vi "Lvi Read Dbl Data Pt.vi"(8 "error in (no error)":errorcluster, 10 "timeout":dbl, 11 "TaskRef":i32) -> (0 "error out":errorcluster, 1 "function return":i32, 2 "DataBuf":dbl, 3 "TaskRef out":i32)   [LabVIEW 2016, in "DtLvLink.lvlib"]
doc: "Calls directly into the entry points of the DLL of the Data Acq SDK to return data points (double data type) from the specified task. This VI is used by the higher-level VI, DtOLRead."
uses:
  <userlib>/LV-Link3/DtLvLink.lvlib
  <userlib>/LV-Link3/DtLvLink_32.dll
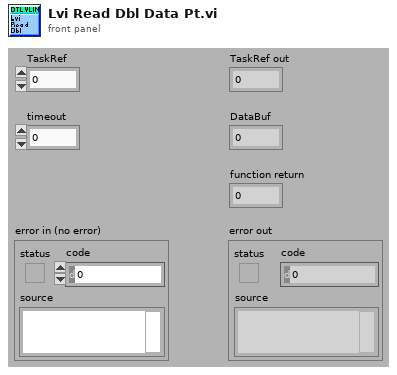
[diagram p1: front panel]
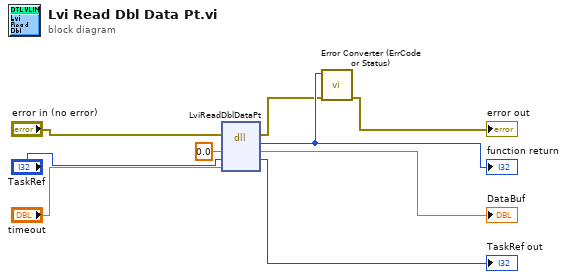
[diagram p0: block diagram]
diagram:
  n1 = dll-call lib="C:/Program Files (x86)/National Instruments/LabVIEW 2016/user.lib/LV-Link3/DtLvLink_32.*" fn="LviReadDblDataPt"(error in="error in (no error)", "DataBuf"=0.0, "TaskRef"="TaskRef", "timeout"="timeout") -> (error out=w2:errorcluster, w9:i32, "DataBuf"=→"DataBuf":dbl, "TaskRef"=→"TaskRef out":i32)  [unwired: 3 in, 1 out]
  "function return" <- w9
  n2 = call <userlib>:"Error Converter (ErrCode or Status).vi"("error in (no error)"=w2, "error code"=w9) -> ("error out"=→"error out":errorcluster)  [unwired: 9 in]
